vi "ExportChannelDataToFile.vi"(4 "error in (no error)":errorcluster, 6 "fileName":string, 7 "axis in":cluster{"keyHandle":u32, "nodeId":u16}={"keyHandle"=0, "nodeId"=1}) -> (0 "error out":errorcluster, 3 "axis out":cluster{"keyHandle":u32, "nodeId":u16}={"keyHandle"=0, "nodeId"=1})   [LabVIEW 2018]
doc: "<B>ExportChannelDataToFile</B> saves data points in a file (File endings: *.csv, *.txt or *.rda)."
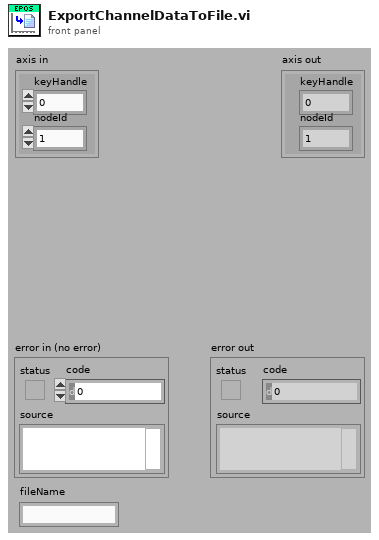
[diagram p1: front panel]
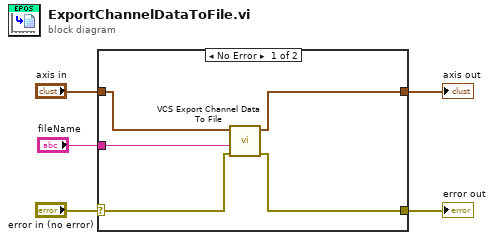
[diagram p0: block diagram]
diagram:
  n1 = case shown="No Error" "error in (no error)" {
    selector: "error in (no error)" -> [w8 w12]
    tunnel: [w9 w12] -> w4
    tunnel: [w10 w11] -> w3
    tunnel: "axis in" -> [w7 w11]
    tunnel: "fileName" -> [w6 _]
    frame No Error {
      n2 = call "VCS Export Channel Data To File.vi"("error in (no error)"=w8, "fileName"=w6, "axis in"=w7) -> ("error out"=w9:errorcluster, "axis out"=w10:cluster{"keyHandle":u32, "nodeId":u16})  [unwired: 7 in]
    }
    frame Error {
    }
  }
  "error out" <- w4
  "axis out" <- w3
